vi "Add Plugin.vi"(8 "error in (no error)":errorcluster, 10 "Plugin":refnum<class "Plugin.lvclass">, 11 "Framework in":refnum<class "Framework.lvclass">) -> (0 "error out":errorcluster, 3 "Framework out":refnum<class "Framework.lvclass">)   [LabVIEW 2016, in "Framework.lvclass"]
uses:
  Framework.lvclass
  Plugin/Plugin.lvclass
  Framework.lvclass/Framework.ctl
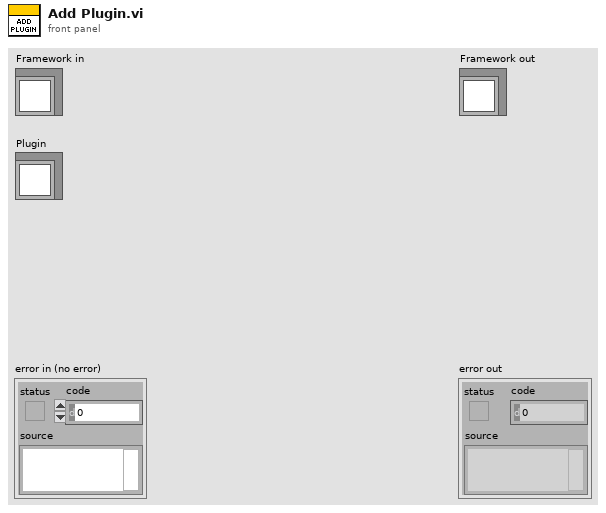
[diagram p1: front panel]
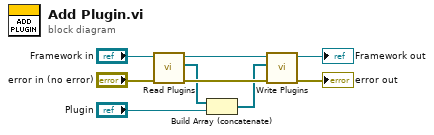
[diagram p0: block diagram]
diagram:
  n1 = call "Read Plugins.vi"("error in (no error)"="error in (no error)", "Framework in"="Framework in") -> ("error out"=w6:errorcluster, "Plugins"=w2:refnum<class "Plugin.lvclass">[], "Framework out"=w7:refnum<class "Framework.lvclass">)  [unwired: 7 in]
  n2 = Build Array (concatenate)(w2, "Plugin") -> (w1:refnum<class "Plugin.lvclass">[])
  n3 = call "Write Plugins.vi"("error in (no error)"=w6, "Plugins"=w1, "Framework in"=w7) -> ("error out"=→"error out":errorcluster, "Framework out"=→"Framework out":refnum<class "Framework.lvclass">)  [unwired: 7 in]
